vi "OpenCVLib_ContainsFace.vi"(8 "error in (no error)":errorcluster, 11 "Image Src":T1) -> (0 "error out":errorcluster, 2 "containsFace":i8, 3 "Image Dst Out":T1)   [LabVIEW 2019]
uses:
  <vilib>/vision/Image Controls.llb/IMAQ Image.ctl
  Binaries/Release/niopencvwrapper.dll
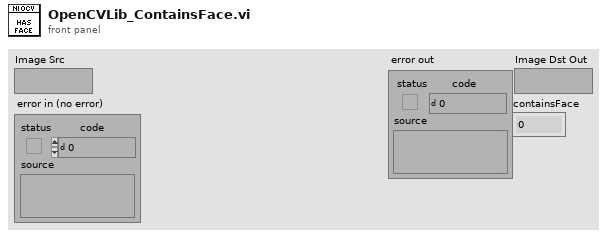
[diagram p1: front panel]
types:
  T1 = typedef "IMAQ Image.ctl" = refnum<image>
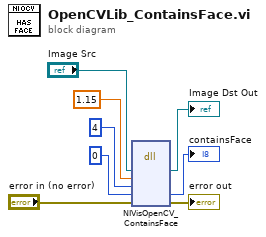
[diagram p0: block diagram]
diagram:
  n1 = dll-call lib="E:/Licenta/trip-validation-system/Binaries/Release/niopencvwrapper.dll" fn="NIVisOpenCV_ContainsFace"("Image Src"="Image Src", "scaleFactor"=1.15, "minNeighbors"=4, "containsFace"=i8 0, "error"="error in (no error)") -> ("Image Src"=→"Image Dst Out":T1, "containsFace"=→"containsFace":i8, "error"=→"error out":errorcluster)  [unwired: 6 in, 2 out]
